vi "QueryInternalTemp.vi"() -> ()   [LabVIEW 2009]
panel:
  out "reference out 4":refnum<visa-resource-name>
  out "error out 2":errorcluster
  in  "reference out 3":refnum<visa-resource-name>
  in  "error out":errorcluster
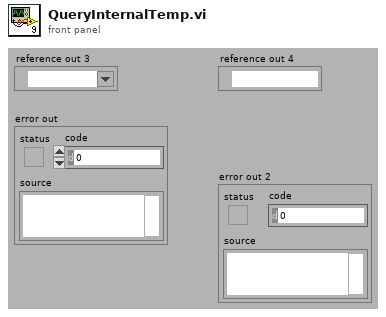
[diagram p1: front panel]
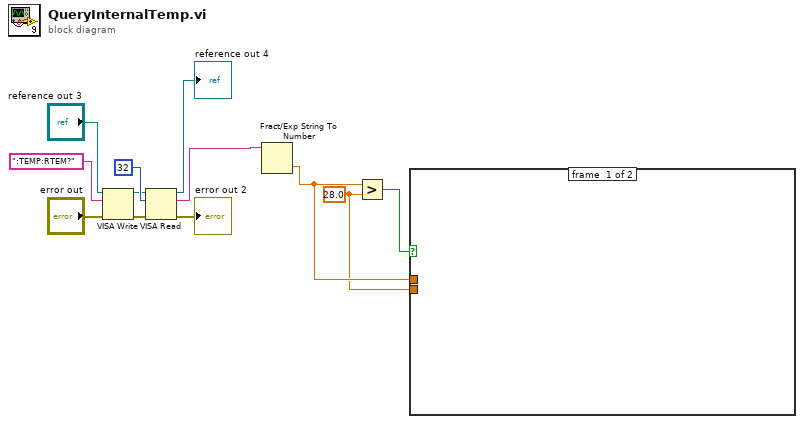
[diagram p0: block diagram]
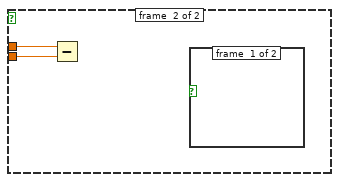
[diagram p2: hidden frame]
diagram:
  w1 = 28.0 ("y")
  n1 = VISA Write(VISA resource name="reference out 3", write buffer=":TEMP:RTEM?", error in (no error)="error out") -> (VISA resource name out=w7:refnum<visa-resource-name>, error out=w6:errorcluster)  [unwired: 1 out]
  n2 = VISA Read(VISA resource name=w7, byte count=u32 32, error in (no error)=w6) -> (VISA resource name out=→"reference out 4":refnum<visa-resource-name>, read buffer=w4:string, error out=→"error out 2":errorcluster)  [unwired: 1 out]
  n3 = Fract/Exp String To Number(string=w4) -> (number=w2:dbl)  [unwired: 3 in, 1 out]
  n4 = Greater?(x=w2, y=w1) -> (0:w3:bool)
  n5 = case shown="True" w3 {
    tunnel: w2 -> [_ w14]
    tunnel: w1 -> [_ w13]
    frame #0 {
    }
    frame #1 {
      n6 = Subtract(x=w14, y=w13) -> ()  [unwired: 1 out]
      n7 = case shown="True" {
        selector: _ -> [_ _]
        frame #0 {
        }
        frame #1 {
        }
      }
    }
  }
